vi "Camera.vi"(0 "Camera in":refnum<class "Camera.lvclass">, 1 "Machine Vision":T4, 2 "Material":T1, 3 "Loop 0":bool, 5 "Stop":bool, 9 "BCG Image Processing":T3={"Brightness"=128.0, "Contrast"=45.0, "Gamma"=1.0} {"Brightness" scale=0.0..400.0; "Contrast" scale=0.0..90.0; "Gamma" scale=0.005..5.0}, 11 "error in (no error)":errorcluster, 12 "Camera settings":T2={"Gamma"=1.0, "Gain"=50, "Sharpness"=0, "Contrast"=0.5, "Exposure"=0.0078125} {"Exposure" min=0.000244140625 max=0.5 scale=0.0002..0.5; "Contrast" min=0.0 max=1.0 scale=0.001..1.0; "Sharpness" min=0 max=2 step=1 scale=0.0..2.0; "Gain" min=0 max=100 step=1 scale=0.1..100.0; "Gamma" min=0.01 max=10.0 scale=0.01..10.0}, 14 "Override presets":bool) -> (4 "Camera out":refnum<class "Camera.lvclass">, 8 "Image":T5(plugin-control), 10 "Camera":dbl[](array[numeric]), 15 "error out":errorcluster)   [LabVIEW 2019, in "Camera.lvclass"]
uses:
  Camera.lvclass
  Machine Vision.ctl
  Image processing.ctl
  Camera settings.ctl
  Material.ctl
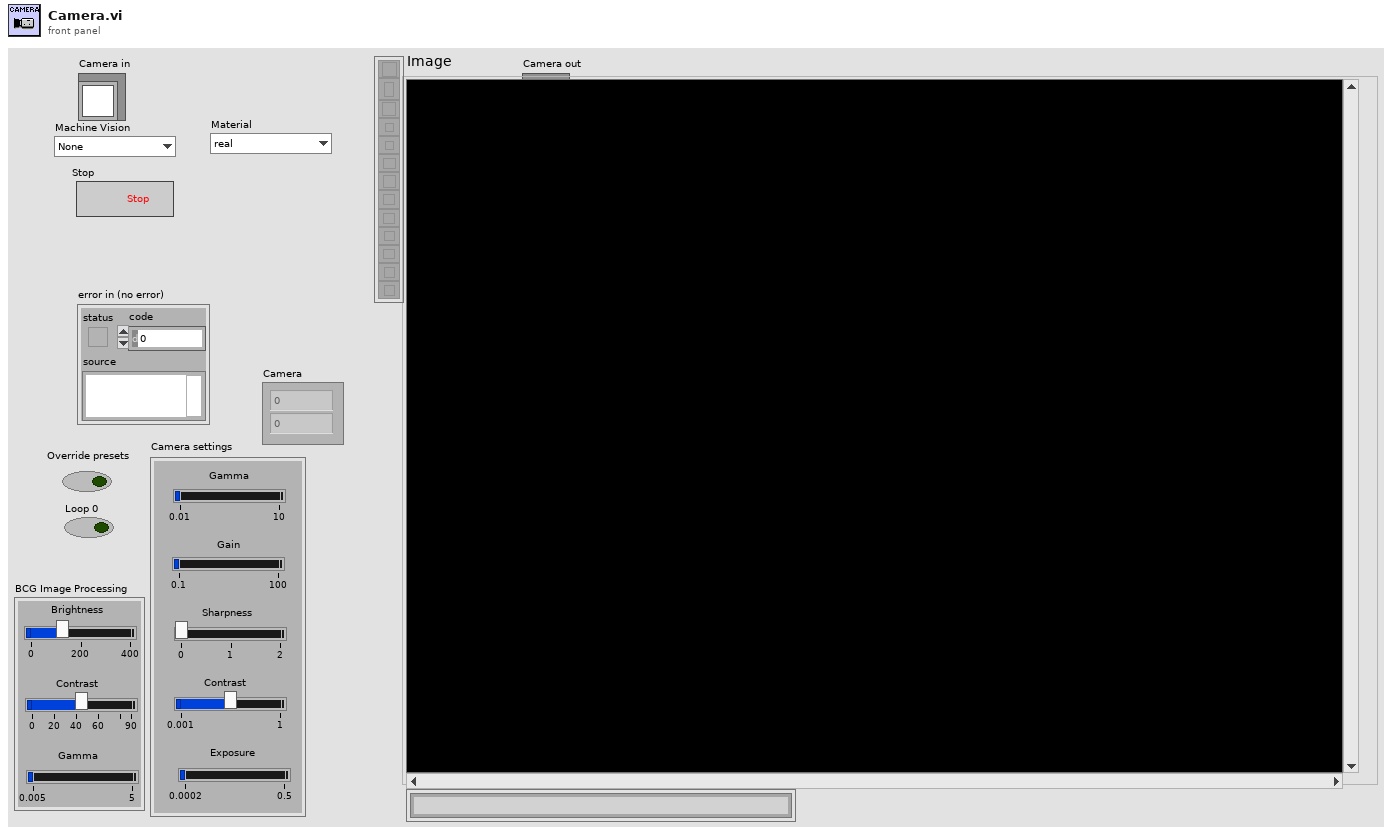
[diagram p1: front panel]
types:
  T1 = typedef "Camera.lvclass/Material.ctl" = enum16{"real", "dummy", "PETG"}
  T2 = typedef "Camera.lvclass/Camera settings.ctl" = cluster{"Gamma":dbl, "Gain":i64, "Sharpness":i64, "Contrast":dbl, "Exposure":dbl}
  T3 = typedef "Camera.lvclass/Image processing.ctl" = cluster{"Brightness":sgl, "Contrast":sgl, "Gamma":sgl}
  T4 = typedef "Camera.lvclass/Machine Vision.ctl" = enum16{"None", "Tray Fiducials", "HPK Silicon", "Hexaboard", "Corner (TL, BR)", "Corner (BL, TR)", "sensor TL", "sensor BL", "sensor TR", "sensor BR", "hexaboard TL", "hexaboard BL", "hexaboard TR", "hexaboard BR"}
  T5 = typedef "IMAQ Image.ctl" = refnum<image>
  T6 = cluster{"Center (Pixels)":cluster{"X":sgl, "Y":sgl}, "Radius (Pixels)":dbl, "Center (Real-World)":cluster{"X":sgl, "Y":sgl}, "Radius (Real-World)":dbl, "Roundness (Real-World)":dbl, "Average Strength":dbl, "Average SNR (dB)":dbl}
  T7 = cluster{"output string":sgl, "output string":sgl}
  T8 = typedef "ROI Descriptor" = cluster{"Global Rectangle":i32[], "Contours":cluster{"ID":enum32{"External", "Internal"}, "Type":u32, "Coordinates":i32[]}[]}
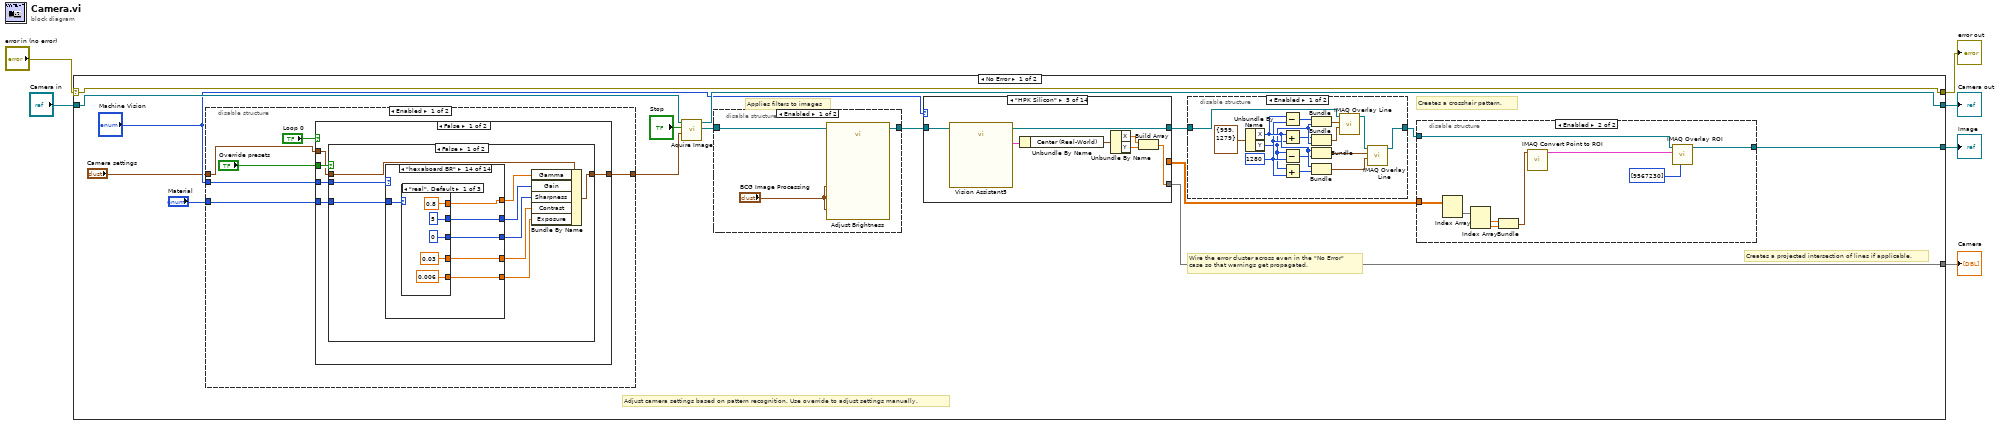
[diagram p0: block diagram]
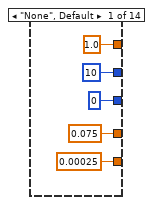
[diagram p2: hidden frame]
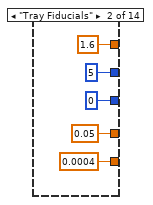
[diagram p3: hidden frame]
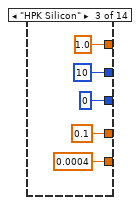
[diagram p4: hidden frame]
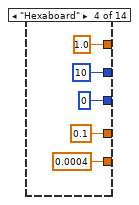
[diagram p5: hidden frame]
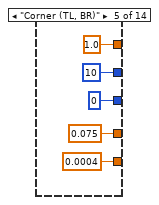
[diagram p6: hidden frame]
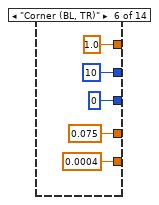
[diagram p7: hidden frame]
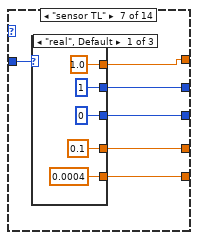
[diagram p8: hidden frame]
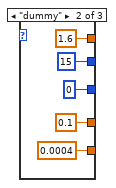
[diagram p9: hidden frame]
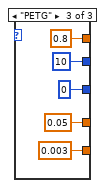
[diagram p10: hidden frame]
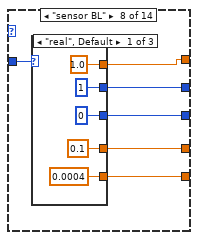
[diagram p11: hidden frame]
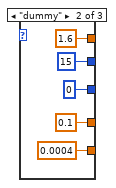
[diagram p12: hidden frame]
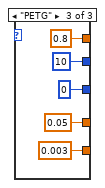
[diagram p13: hidden frame]
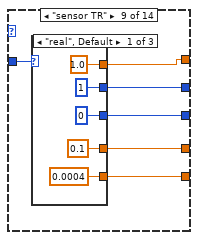
[diagram p14: hidden frame]
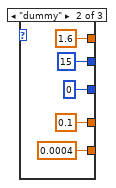
[diagram p15: hidden frame]
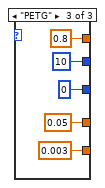
[diagram p16: hidden frame]
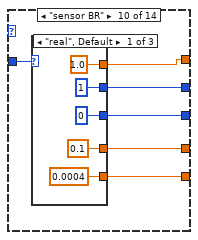
[diagram p17: hidden frame]
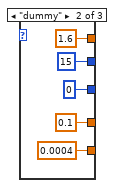
[diagram p18: hidden frame]
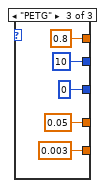
[diagram p19: hidden frame]
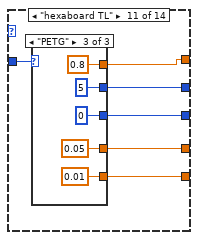
[diagram p20: hidden frame]
diagram:
  n1 = case shown="No Error" "error in (no error)" {
    selector: "error in (no error)" -> [w21 w352]
    tunnel: [w21 w352] -> w5
    tunnel: [w19 w351] -> w4
    tunnel: "Camera in" -> [w20 w351]
    tunnel: [w18 _] -> w2
    tunnel: [w15 _] -> w1
    frame No Error {
      # "Applies filters to images"
      # "Adjust camera settings based on pattern recognition. Use override to adjust settings manually."
      # "Creates a projected intersection of lines if applicable."
      # "Creates a crosshair pattern."
      # "Wire the error cluster across even in the \"No Error\"\ncase so that warnings get propagated."
      n2 = disable-structure shown="Enabled" {
        disable-tunnel: "Machine Vision" -> [w27 _]
        disable-tunnel: "Camera settings" -> [w26 w248]
        disable-tunnel: [w25 w248] -> w8
        disable-tunnel: "Material" -> [w22 _]
        frame Enabled {
          n3 = case shown="False" "Loop 0" {
            tunnel: "Override presets" -> [w32 _]
            tunnel: w27 -> [w31 _]
            tunnel: w26 -> [w30 w247]
            tunnel: [w29 w246] -> w25
            tunnel: w22 -> [w28 _]
            frame False {
              n4 = case shown="False" w32 {
                tunnel: w31 -> [w41 _]
                tunnel: w30 -> [w40 w240]
                tunnel: [w34 w240] -> w29
                tunnel: w28 -> [w33 _]
                frame False {
                  n5 = case shown="\"hexaboard BR\"" w41 {
                    tunnel: [1.0 ("Gamma::Value") 1.6 ("Gamma::Value") 1.0 ("Gamma::Value") 1.0 ("Gamma::Value") 1.0 ("Gamma::Value") 1.0 ("Gamma::Value") w76 w98 w119 w140 w156 w177 w198 w219] -> w39
                    tunnel: [i64 10 ("Gain::Value") i64 5 ("Gain::Value") i64 10 ("Gain::Value") i64 10 ("Gain::Value") i64 10 ("Gain::Value") i64 10 ("Gain::Value") w75 w97 w118 w139 w157 w178 w199 w220] -> w38
                    tunnel: [i64 0 ("Sharpness::Value") i64 0 ("Sharpness::Value") i64 0 ("Sharpness::Value") i64 0 ("Sharpness::Value") i64 0 ("Sharpness::Value") i64 0 ("Sharpness::Value") w74 w96 w117 w138 w158 w179 w200 w221] -> w37
                    tunnel: [0.075 ("Contrast::Value") 0.05 ("Contrast::Value") 0.1 ("Contrast::Value") 0.1 ("Contrast::Value") 0.075 ("Contrast::Value") 0.075 ("Contrast::Value") w73 w95 w116 w137 w159 w180 w201 w222] -> w36
                    tunnel: [0.00025 ("Exposure::Value") 0.0004 ("Exposure::Value") 0.0004 ("Exposure::Value") 0.0004 ("Exposure::Value") 0.0004 ("Exposure::Value") 0.0004 ("Exposure::Value") w72 w94 w115 w136 w160 w181 w202 w223] -> w35
                    tunnel: w33 -> [_ _ _ _ _ _ w77 w93 w114 w135 w161 w182 w203 w224]
                    frame "None", Default {
                    }
                    frame "Tray Fiducials" {
                    }
                    frame "HPK Silicon" {
                    }
                    frame "Hexaboard" {
                    }
                    frame "Corner (TL, BR)" {
                    }
                    frame "Corner (BL, TR)" {
                    }
                    frame "sensor TL" {
                      n6 = case shown="\"real\", Default" w77 {
                        tunnel: [1.0 ("Gamma::Value") 1.6 ("Gamma::Value") 0.8 ("Gamma::Value")] -> w76
                        tunnel: [0.1 ("Contrast::Value") 0.1 ("Contrast::Value") 0.05 ("Contrast::Value")] -> w73
                        tunnel: [i64 0 ("Sharpness::Value") i64 0 ("Sharpness::Value") i64 0 ("Sharpness::Value")] -> w74
                        tunnel: [i64 1 ("Gain::Value") i64 15 ("Gain::Value") i64 10 ("Gain::Value")] -> w75
                        tunnel: [0.0004 ("Exposure::Value") 0.0004 ("Exposure::Value") 0.003 ("Exposure::Value")] -> w72
                        frame "real", Default {
                        }
                        frame "dummy" {
                        }
                        frame "PETG" {
                        }
                      }
                    }
                    frame "sensor BL" {
                      n7 = case shown="\"real\", Default" w93 {
                        tunnel: [1.0 ("Gamma::Value") 1.6 ("Gamma::Value") 0.8 ("Gamma::Value")] -> w98
                        tunnel: [0.1 ("Contrast::Value") 0.1 ("Contrast::Value") 0.05 ("Contrast::Value")] -> w95
                        tunnel: [i64 0 ("Sharpness::Value") i64 0 ("Sharpness::Value") i64 0 ("Sharpness::Value")] -> w96
                        tunnel: [i64 1 ("Gain::Value") i64 15 ("Gain::Value") i64 10 ("Gain::Value")] -> w97
                        tunnel: [0.0004 ("Exposure::Value") 0.0004 ("Exposure::Value") 0.003 ("Exposure::Value")] -> w94
                        frame "real", Default {
                        }
                        frame "dummy" {
                        }
                        frame "PETG" {
                        }
                      }
                    }
                    frame "sensor TR" {
                      n8 = case shown="\"real\", Default" w114 {
                        tunnel: [1.0 ("Gamma::Value") 1.6 ("Gamma::Value") 0.8 ("Gamma::Value")] -> w119
                        tunnel: [0.1 ("Contrast::Value") 0.1 ("Contrast::Value") 0.05 ("Contrast::Value")] -> w116
                        tunnel: [i64 0 ("Sharpness::Value") i64 0 ("Sharpness::Value") i64 0 ("Sharpness::Value")] -> w117
                        tunnel: [i64 1 ("Gain::Value") i64 15 ("Gain::Value") i64 10 ("Gain::Value")] -> w118
                        tunnel: [0.0004 ("Exposure::Value") 0.0004 ("Exposure::Value") 0.003 ("Exposure::Value")] -> w115
                        frame "real", Default {
                        }
                        frame "dummy" {
                        }
                        frame "PETG" {
                        }
                      }
                    }
                    frame "sensor BR" {
                      n9 = case shown="\"real\", Default" w135 {
                        tunnel: [1.0 ("Gamma::Value") 1.6 ("Gamma::Value") 0.8 ("Gamma::Value")] -> w140
                        tunnel: [0.1 ("Contrast::Value") 0.1 ("Contrast::Value") 0.05 ("Contrast::Value")] -> w137
                        tunnel: [i64 0 ("Sharpness::Value") i64 0 ("Sharpness::Value") i64 0 ("Sharpness::Value")] -> w138
                        tunnel: [i64 1 ("Gain::Value") i64 15 ("Gain::Value") i64 10 ("Gain::Value")] -> w139
                        tunnel: [0.0004 ("Exposure::Value") 0.0004 ("Exposure::Value") 0.003 ("Exposure::Value")] -> w136
                        frame "real", Default {
                        }
                        frame "dummy" {
                        }
                        frame "PETG" {
                        }
                      }
                    }
                    frame "hexaboard TL" {
                      n10 = case shown="\"PETG\"" w161 {
                        tunnel: [0.006 ("Exposure::Value") 0.006 ("Exposure::Value") 0.01 ("Exposure::Value")] -> w160
                        tunnel: [0.03 ("Contrast::Value") 0.03 ("Contrast::Value") 0.05 ("Contrast::Value")] -> w159
                        tunnel: [i64 0 ("Sharpness::Value") i64 0 ("Sharpness::Value") i64 0 ("Sharpness::Value")] -> w158
                        tunnel: [i64 5 ("Gain::Value") i64 5 ("Gain::Value") i64 5 ("Gain::Value")] -> w157
                        tunnel: [0.8 ("Gamma::Value") 0.8 ("Gamma::Value") 0.8 ("Gamma::Value")] -> w156
                        frame "real", Default {
                        }
                        frame "dummy" {
                        }
                        frame "PETG" {
                        }
                      }
                    }
                    frame "hexaboard BL" {
                      n11 = case shown="\"PETG\"" w182 {
                        tunnel: [0.006 ("Exposure::Value") 0.006 ("Exposure::Value") 0.01 ("Exposure::Value")] -> w181
                        tunnel: [0.03 ("Contrast::Value") 0.03 ("Contrast::Value") 0.05 ("Contrast::Value")] -> w180
                        tunnel: [i64 0 ("Sharpness::Value") i64 0 ("Sharpness::Value") i64 0 ("Sharpness::Value")] -> w179
                        tunnel: [i64 5 ("Gain::Value") i64 5 ("Gain::Value") i64 5 ("Gain::Value")] -> w178
                        tunnel: [0.8 ("Gamma::Value") 0.8 ("Gamma::Value") 0.8 ("Gamma::Value")] -> w177
                        frame "real", Default {
                        }
                        frame "dummy" {
                        }
                        frame "PETG" {
                        }
                      }
                    }
                    frame "hexaboard TR" {
                      n12 = case shown="\"PETG\"" w203 {
                        tunnel: [0.006 ("Exposure::Value") 0.006 ("Exposure::Value") 0.01 ("Exposure::Value")] -> w202
                        tunnel: [0.03 ("Contrast::Value") 0.03 ("Contrast::Value") 0.05 ("Contrast::Value")] -> w201
                        tunnel: [i64 0 ("Sharpness::Value") i64 0 ("Sharpness::Value") i64 0 ("Sharpness::Value")] -> w200
                        tunnel: [i64 5 ("Gain::Value") i64 5 ("Gain::Value") i64 5 ("Gain::Value")] -> w199
                        tunnel: [0.8 ("Gamma::Value") 0.8 ("Gamma::Value") 0.8 ("Gamma::Value")] -> w198
                        frame "real", Default {
                        }
                        frame "dummy" {
                        }
                        frame "PETG" {
                        }
                      }
                    }
                    frame "hexaboard BR" {
                      n13 = case shown="\"real\", Default" w224 {
                        tunnel: [0.006 ("Exposure::Value") 0.006 ("Exposure::Value") 0.01 ("Exposure::Value")] -> w223
                        tunnel: [0.03 ("Contrast::Value") 0.03 ("Contrast::Value") 0.05 ("Contrast::Value")] -> w222
                        tunnel: [i64 0 ("Sharpness::Value") i64 0 ("Sharpness::Value") i64 0 ("Sharpness::Value")] -> w221
                        tunnel: [i64 5 ("Gain::Value") i64 5 ("Gain::Value") i64 5 ("Gain::Value")] -> w220
                        tunnel: [0.8 ("Gamma::Value") 0.8 ("Gamma::Value") 0.8 ("Gamma::Value")] -> w219
                        frame "real", Default {
                        }
                        frame "dummy" {
                        }
                        frame "PETG" {
                        }
                      }
                    }
                  }
                  n14 = Bundle By Name(cluster=w40, "Gamma"=w39, "Gain"=w38, "Sharpness"=w37, "Contrast"=w36, "Exposure"=w35) -> (w34:T2)
                }
                frame True {
                }
              }
            }
            frame True {
              n15 = Bundle By Name(cluster=w247, "Gamma"=0.0, "Gain"=i64 0, "Sharpness"=i64 0, "Contrast"=0.0, "Exposure"=0.0) -> (w246:T2)
            }
          }
        }
        frame Disabled {
        }
      }
      n16 = call-dynamic "Aquire Image.vi"("Cluster"=w8, "Stop"="Stop", "Camera in"=w20) -> ("Image Out"=w13:T5, "Camera out"=w19:refnum<class "Camera.lvclass">)  [unwired: 6 in, 1 out]
      n17 = disable-structure shown="Enabled" {
        disable-tunnel: w13 -> [w251 w252]
        disable-tunnel: [w250 w252] -> w12
        frame Enabled {
          n18 = call "Adjust Brightness"("Image In"=w251, "Red BCG Values (Brightness 1)"="BCG Image Processing", "Green BCG Values (Brightness 1)"="BCG Image Processing", "Blue BCG Values (Brightness 1)"="BCG Image Processing") -> ("Image Out"=w250:T5)  [unwired: 22 in, 1 out]
        }
        frame Disabled {
        }
      }
      n19 = case shown="\"HPK Silicon\"" "Machine Vision" {
        tunnel: [w281 w286 w294 w299 w304 w311 w317 w321 w326 w331 w336 w341 w346 _] -> w18
        tunnel: [w284 w287 w297 w302 w306 w313 w316 w323 w328 w333 w338 w343 w348 w350] -> w17
        tunnel: w12 -> [w285 w288 w296 w301 w305 w314 w319 w324 w329 w334 w339 w344 w349 w350]
        tunnel: [_ _ w293 w298 _ w310 w315 w320 w325 w330 w335 w340 w345 _] -> w14
        frame "Tray Fiducials" {
          n20 = call "Vision Assistant"("Image In"=w285) -> ("Image Out"=w284:T5, "Fitted Circle (Find Circular Edge 1)"=w280:T6)  [unwired: 24 in, 1 out]
          n21 = Unbundle By Name(w280) -> ("Center (Real-World)"=w283:cluster{"X":sgl, "Y":sgl})
          n22 = Unbundle By Name(w283) -> ("X"=w282:sgl, "Y"=w279:sgl)
          n23 = Build Array(w282, w279) -> (w281:sgl[])
        }
        frame "Hexaboard" {
          n24 = call "Vision Assistant2"("Image In"=w288) -> ("Image Out"=w287:T5, "Fitted Circle (Find Circular Edge 1)"=w290:T6)  [unwired: 24 in, 1 out]
          n25 = Unbundle By Name(w290) -> ("Center (Real-World)"=w292:cluster{"X":sgl, "Y":sgl})
          n26 = Unbundle By Name(w292) -> ("X"=w291:sgl, "Y"=w289:sgl)
          n27 = Build Array(w291, w289) -> (w286:sgl[])
        }
        frame "Corner (TL, BR)" {
          n28 = call "Vision Assistant3"("Image In"=w296) -> ("Image Out"=w297:T5, "Caliper Results (Top Left, Bottom Right)"=w293:sgl[][], "Calibrated Results (Top Left, Bottom Right)"=w295:sgl[][])  [unwired: 23 in, 1 out]
          n29 = Index Array(array=w295) -> (element=w294:sgl[])  [unwired: 2 in]
        }
        frame "Corner (BL, TR)" {
          n30 = call "Vision Assistant4"("Image In"=w301) -> ("Image Out"=w302:T5, "Caliper Results (Bottom Left, Top Right)"=w298:sgl[][], "Calibrated Results (Bottom Left, Top Right)"=w300:sgl[][])  [unwired: 23 in, 1 out]
          n31 = Index Array(array=w300) -> (element=w299:sgl[])  [unwired: 2 in]
        }
        frame "HPK Silicon" {
          n32 = call "Vision Assistant5"("Image In"=w305) -> ("Image Out"=w306:T5, "Fitted Circle (Find Circular Edge 1)"=w303:T6)  [unwired: 24 in, 1 out]
          n33 = Unbundle By Name(w303) -> ("Center (Real-World)"=w309:cluster{"X":sgl, "Y":sgl})
          n34 = Unbundle By Name(w309) -> ("X"=w308:sgl, "Y"=w307:sgl)
          n35 = Build Array(w308, w307) -> (w304:sgl[])
        }
        frame "sensor TL" {
          n36 = call "Vision Assistant6"("Image In"=w314) -> ("Image Out"=w313:T5, "Caliper Results (Caliper 1)"=w310:sgl[][], "Calibrated Results (Caliper 1)"=w312:sgl[][])  [unwired: 23 in, 1 out]
          n37 = Index Array(array=w312) -> (element=w311:sgl[])  [unwired: 2 in]
        }
        frame "sensor BL" {
          n38 = call "Vision Assistant7"("Image In"=w319) -> ("Image Out"=w316:T5, "Caliper Results (Caliper 1)"=w315:sgl[][], "Calibrated Results (Caliper 1)"=w318:sgl[][])  [unwired: 23 in, 1 out]
          n39 = Index Array(array=w318) -> (element=w317:sgl[])  [unwired: 2 in]
        }
        frame "sensor TR" {
          n40 = call "Vision Assistant8"("Image In"=w324) -> ("Image Out"=w323:T5, "Caliper Results (Caliper 1)"=w320:sgl[][], "Calibrated Results (Caliper 1)"=w322:sgl[][])  [unwired: 23 in, 1 out]
          n41 = Index Array(array=w322) -> (element=w321:sgl[])  [unwired: 2 in]
        }
        frame "sensor BR" {
          n42 = call "Vision Assistant9"("Image In"=w329) -> ("Image Out"=w328:T5, "Caliper Results (Caliper 1)"=w325:sgl[][], "Calibrated Results (Caliper 1)"=w327:sgl[][])  [unwired: 23 in, 1 out]
          n43 = Index Array(array=w327) -> (element=w326:sgl[])  [unwired: 2 in]
        }
        frame "hexaboard TL" {
          n44 = call "Vision Assistant18"("Image In"=w334) -> ("Image Out"=w333:T5, "Caliper Results (Caliper 1)"=w330:sgl[][], "Calibrated Results (Caliper 1)"=w332:sgl[][])  [unwired: 23 in, 1 out]
          n45 = Index Array(array=w332) -> (element=w331:sgl[])  [unwired: 2 in]
        }
        frame "hexaboard BL" {
          n46 = call "Vision Assistant11"("Image In"=w339) -> ("Image Out"=w338:T5, "Caliper Results (Caliper 1)"=w335:sgl[][], "Calibrated Results (Caliper 1)"=w337:sgl[][])  [unwired: 23 in, 1 out]
          n47 = Index Array(array=w337) -> (element=w336:sgl[])  [unwired: 2 in]
        }
        frame "hexaboard TR" {
          n48 = call "Vision Assistant12"("Image In"=w344) -> ("Image Out"=w343:T5, "Caliper Results (Caliper 1)"=w340:sgl[][], "Calibrated Results (Caliper 1)"=w342:sgl[][])  [unwired: 23 in, 1 out]
          n49 = Index Array(array=w342) -> (element=w341:sgl[])  [unwired: 2 in]
        }
        frame "hexaboard BR" {
          n50 = call "Vision Assistant13"("Image In"=w349) -> ("Image Out"=w348:T5, "Caliper Results (Caliper 1)"=w345:sgl[][], "Calibrated Results (Caliper 1)"=w347:sgl[][])  [unwired: 23 in, 1 out]
          n51 = Index Array(array=w347) -> (element=w346:sgl[])  [unwired: 2 in]
        }
        frame "None", Default {
        }
      }
      n52 = disable-structure shown="Enabled" {
        disable-tunnel: w17 -> [w264 w278]
        disable-tunnel: [w263 w278] -> w16
        frame Enabled {
          w271 = 1280
          n53 = Unbundle By Name(cluster{"X":i32, "Y":i32} {"X"=959, "Y"=1279} ("Cross Hair coordinates")) -> ("X"=w274:i32, "Y"=w270:i32)
          n54 = Subtract(x=w274, y=w271) -> (x-y=w266:i32)
          n55 = Add(x=w274, y=w271) -> (x+y=w267:i32)
          n56 = Subtract(x=w270, y=w271) -> (x-y=w272:i32)
          n57 = Add(x=w270, y=w271) -> (x+y=w273:i32)
          n58 = Bundle(w266, "Y"=w270) -> (w269:cluster{i32, "Y":i32})  [unwired: 1 in]
          n59 = Bundle(w267, "Y"=w270) -> (w268:cluster{i32, "Y":i32})  [unwired: 1 in]
          n60 = Bundle("X"=w274, w272) -> (w275:cluster{"X":i32, i32})  [unwired: 1 in]
          n61 = Bundle("X"=w274, w273) -> (w276:cluster{"X":i32, i32})  [unwired: 1 in]
          n62 = call "IMAQ Overlay Line"("End Point"=w268, "Start Point"=w269, "Image"=w264) -> ("Image Out"=w277:T5)  [unwired: 7 in, 1 out]
          n63 = call "IMAQ Overlay Line"("End Point"=w276, "Start Point"=w275, "Image"=w277) -> ("Image Out"=w263:T5)  [unwired: 7 in, 1 out]
        }
        frame Disabled {
        }
      }
      n64 = disable-structure shown="Enabled" {
        disable-tunnel: [w253 w258] -> w15
        disable-tunnel: w16 -> [w253 w257]
        disable-tunnel: w14 -> [_ w256]
        frame Disabled {
        }
        frame Enabled {
          n65 = Index Array(array=w256) -> (element=w255:sgl[])  [unwired: 2 in]
          n66 = Index Array(array=w255) -> (element #1=w259:sgl, element #2=w261:sgl)  [unwired: 2 in]
          n67 = Bundle("output string"=w259, "output string"=w261) -> (w262:T7)  [unwired: 1 in]
          n68 = call "IMAQ Convert Point to ROI"("Point"=w262) -> ("ROI Descriptor"=w260:T8)  [unwired: 8 in, 1 out]
          n69 = call "IMAQ Overlay ROI"("Colors (Green)"=u32[] [9567230], "ROI Descriptor"=w260, "Image"=w257) -> ("Image Out"=w258:T5)  [unwired: 7 in, 1 out]
        }
      }
    }
    frame Error {
    }
  }
  "error out" <- w5
  "Camera out" <- w4
  "Camera" <- w2
  "Image" <- w1
